vi "READ - FRF File.vi"(0 "reference in":refnum<class "TEXT.lvclass">, 5 "error in (no error)":errorcluster, 7 "TDMS Path - READ":path) -> (14 "reference out":refnum<class "TEXT.lvclass">, 19 "error out":errorcluster)   [LabVIEW 2022 SP3, in "TEXT.lvclass"]
uses:
  TEXT.lvclass
  API/Generic Utilities_class/Generic Utilities.lvclass
  API/GSwFormDSP_class/GSwFormDSP.lvclass
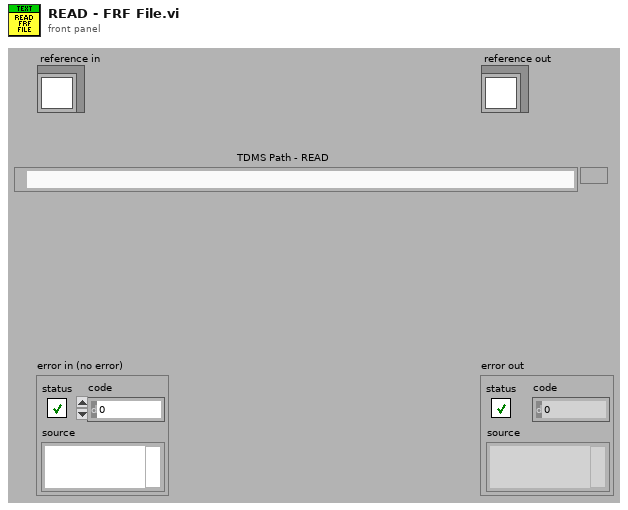
[diagram p1: front panel]
types:
  T1 = typedef "TEXT.lvclass/ObjectAttributesRef.ctl" = refnum<data-value>
  T2 = typedef "TEXT.lvclass/ObjectAttributes.ctl" = cluster{"Time Data":refnum<class "GSwFormDSP.lvclass">, "New Time Data Obj?":bool}
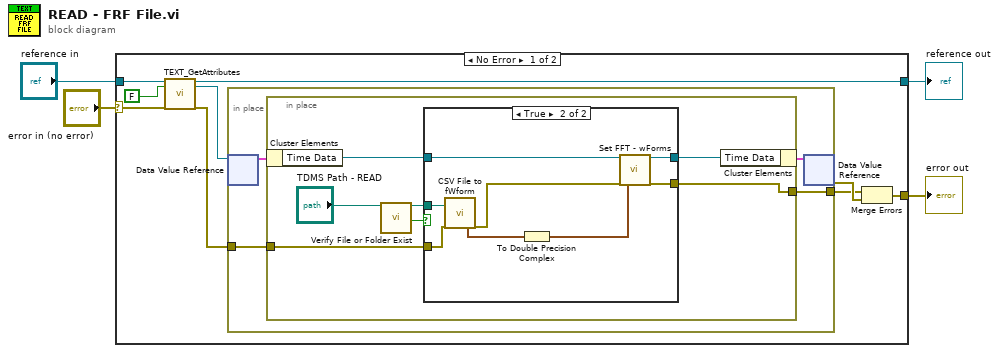
[diagram p0: block diagram]
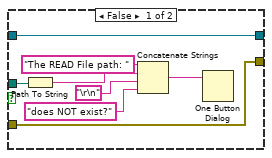
[diagram p2: hidden frame]
diagram:
  n1 = case shown="No Error" "error in (no error)" {
    selector: "error in (no error)" -> [w8 w42]
    tunnel: [w13 w42] -> w3
    tunnel: [w7 w41] -> w1
    tunnel: "reference in" -> [w10 w41]
    frame No Error {
      n2 = call "TEXT_GetAttributes.vi"("reference in"=w10, "return data? (T)"=FALSE, "error in (no error)"=w8) -> ("reference out"=w7:refnum<class "TEXT.lvclass">, "attributes ref"=w6:T1, "error out"=w5:errorcluster)  [unwired: 13 in, 1 out]
      n3 = in-place {
        in-place-border: [w14] -> w11
        in-place-border: w5 -> [w15]
        n4 = in-place-dvr #1(w6) -> (w16:T2)  [unwired: 1 out]
        n5 = in-place {
          in-place-border: w15 -> [w19]
          in-place-border: [w18] -> w14
          n6 = in-place-cluster #2(w16) -> ("Time Data"=w20:refnum<class "GSwFormDSP.lvclass">)
          n7 = call "Verify File or Folder Exist.vi"("path"="TDMS Path - READ") -> ("dup path"=w24:path, "file or folder exists?"=w23:bool)  [unwired: 16 in, 1 out]
          n8 = case shown="True" w23 {
            tunnel: w20 -> [w32 w40]
            tunnel: [w32 w35] -> w21
            tunnel: w24 -> [w30 w39]
            tunnel: w19 -> [w31 w38]
            tunnel: [w31 w34] -> w18
            frame False {
              n9 = Path To String(path=w30) -> (string=w28:string)
              n10 = Concatenate Strings("The READ File path: ", w28, "\r\n", "does NOT exist?") -> (w25:string)
              n11 = One Button Dialog(message=w25) -> ()  [unwired: 1 in, 1 out]
            }
            frame True {
              n12 = call "CSV File to fWform.vi"("CSV Path IN"=w39, "error in (no error)"=w38) -> ("wForms"=w36:waveform(dbl)[], "error out"=w37:errorcluster)  [unwired: 15 in, 1 out]
              n13 = To Double Precision Complex(1:w36) -> (0:w33:waveform(cdb)[])
              n14 = call "Set FFT - wForms.vi"("reference in"=w40, "error in (no error)"=w37, "FFT wForms"=w33) -> ("reference out"=w35:refnum<class "GSwFormDSP.lvclass">, "error out"=w34:errorcluster)  [unwired: 15 in]
            }
          }
          n15 = in-place-cluster #2("Time Data"=w21) -> (w17:T2)
        }
        n16 = in-place-dvr #1(w17) -> (w12:errorcluster)  [unwired: 1 out]
      }
      n17 = Merge Errors(w11, w12) -> (w13:errorcluster)
    }
    frame Error {
    }
  }
  "error out" <- w3
  "reference out" <- w1
